vi "ordering.vi"(2 "Ascend":bool=TRUE, 3 "N_mech":u32=4, 4 "N":u32[](array[numeric])=[1, 1, 1, 1]) -> (1 "Order":u32[](array[numeric]))   [LabVIEW 2019, in "Userlib.lvlib"]
uses:
  Userlib.lvlib
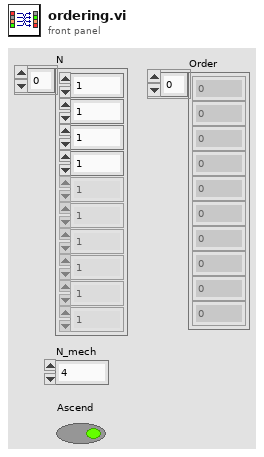
[diagram p1: front panel]
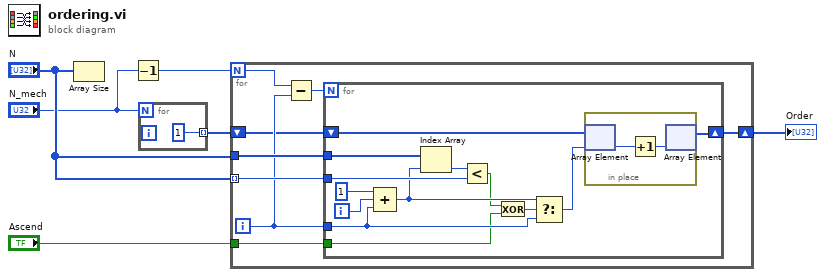
[diagram p0: block diagram]
diagram:
  n1 = Array Size(array="N") -> ()  [unwired: 1 out]
  n2 = Decrement(x="N_mech") -> (x-1=w6:u32)
  n3 = for {
    N: "N_mech" -> [_]
    tunnel: [u32 1 ("y")] -> w5 mode=indexing
  }
  n4 = for {
    N: w6 -> [w12]
    tunnel: "N" -> [w14] mode=indexing
    tunnel: "N" -> [w15]
    shift-right: [w10] -> w3
    shift-left: w5 -> [w9]
    tunnel: "Ascend" -> [w8]
    i -> [w11]
    n5 = Subtract(x=w12, y=w11) -> (x-y=w13:i32)
    n6 = for {
      N: w13 -> [_]
      tunnel: w15 -> [w28]
      tunnel: w14 -> [w26]
      tunnel: w11 -> [w19]
      shift-right: [w22] -> w10
      shift-left: w9 -> [w23]
      tunnel: w8 -> [w16]
      i -> [w25]
      n7 = Compound Arithmetic op=ADD(1 ("y"), w25, w19) -> (w21:i32)
      n8 = Index Array(array=w28, index=w21) -> (element=w27:u32)
      n9 = Less?(x=w27, y=w26) -> (x < y?=w17:bool)
      n10 = Exclusive Or(1:w16, 2:w17) -> (0:w18:bool)
      n11 = Select(t=w21, s=w18, f=w19) -> (s? t:f=w24:i32)
      n12 = in-place {
        n13 = in-place-array #1(w23, w24) -> (w29:u32)
        n14 = Increment(x=w29) -> (x+1=w30:u32)
        n15 = in-place-array #1(w30) -> (w22:u32[])  [unwired: 1 out]
      }
    }
  }
  "Order" <- w3
